vi "GObject_Ref_to_Class_Name.vi"(9 "error in":errorcluster, 10 "GObject Ref In":refnum<vi>) -> (0 "Class Name Out":string, 1 "error out":errorcluster, 2 "GObject Ref Out":refnum<vi>)   [LabVIEW 2012]
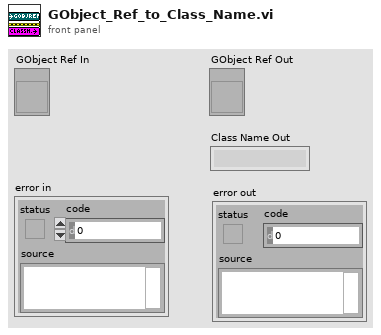
[diagram p1: front panel]
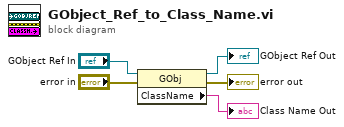
[diagram p0: block diagram]
diagram:
  n1 = property class="GObj"(reference="GObject Ref In", error in="error in") -> (reference out=→"GObject Ref Out":refnum<vi>, error out=→"error out":errorcluster, "ClassName"=→"Class Name Out":string)
